vi "Save To TIFF.vi"(10 "Logging Cluster":T2 {"Exp params"."TSFrames" min=1 step=1; "Exp params"."TSfps" min=0.001 max=90.0 step=0.001 format="%_4g"}, 11 "img dst":T1) -> (3 "Image Out (duplicate)":T1)   [LabVIEW 2020]
uses:
  _controls/Logging Cluster.ctl
  _controls/Exp Params.ctl
  <vilib>/vision/Image Controls.llb/IMAQ Image.ctl
  _globals/OpticalPrime Controls.vi
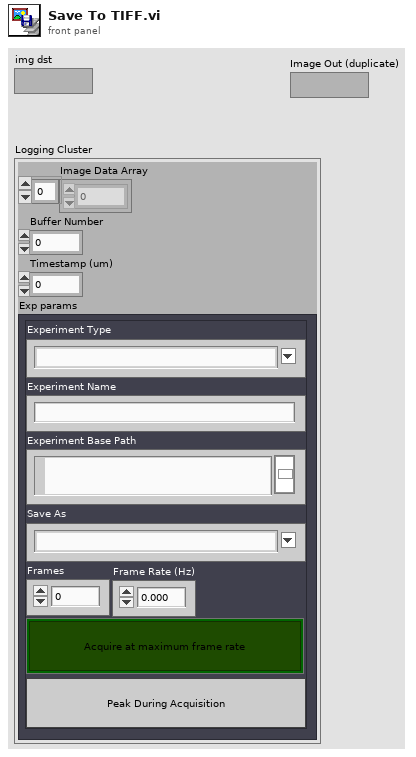
[diagram p1: front panel]
types:
  T1 = typedef "IMAQ Image.ctl" = refnum<image>
  T2 = typedef "Logging Cluster.ctl" = cluster{"Image Data Array":u8[], "Buffer Number":i32, "Timestamp (um)":u64, "Exp params":T3}
  T3 = typedef "Exp Params.ctl" = cluster{"Experiment Type":string, "Experiment Name":string, "ExpPath":path, "Save As":string, "TSFrames":i32, "TSfps":dbl, "Streaming":bool, "tdms ref":refnum<k34>, "frame #":i64, "Full Path":path, "PeakOnQueue":bool}
  T4 = enum16{"open", "replace", "create", "open or create", "replace or create", "replace or create with confirmation"}
  T5 = typedef "xiCam.ctl" = cluster{"Exposure Time (ms)":u32, "cam0 Session":T6, "Camera ROI":cluster{"Width":u32, "Height":u32, "Offset X":u32, "Offset Y":u32}, "Command":string}
  T6 = typedef "IMAQdx.ctl" = refnum<k21>
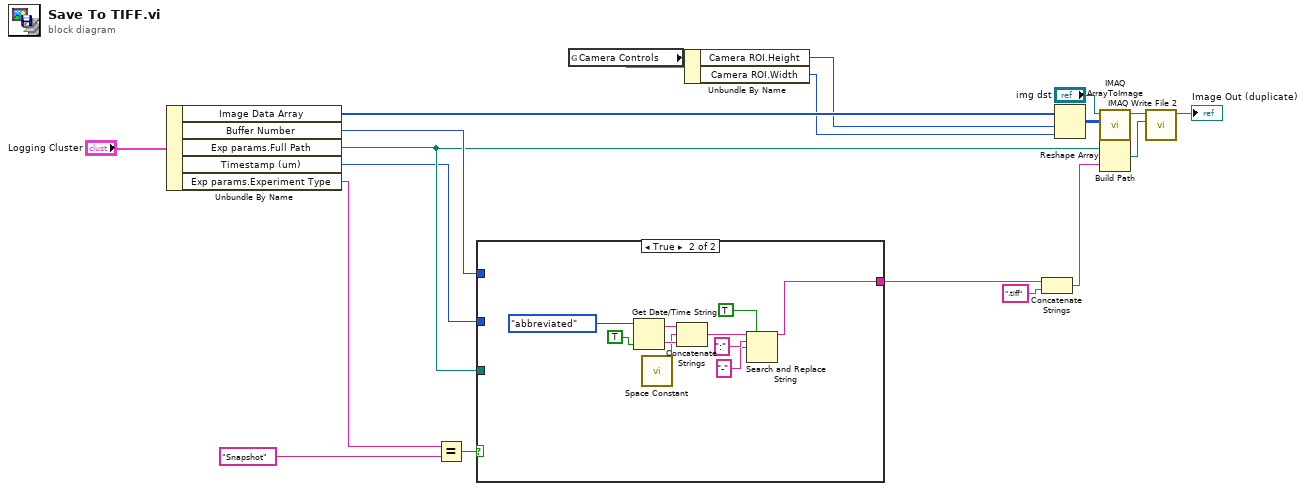
[diagram p0: block diagram]
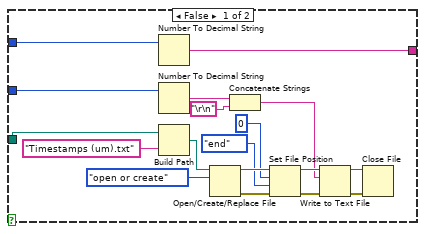
[diagram p2: hidden frame]
diagram:
  n1 = Unbundle By Name("Logging Cluster") -> ("Image Data Array"=w14:u8[], "Buffer Number"=w19:i32, "Exp params.Full Path"=w12:path, "Timestamp (um)"=w11:u64, "Exp params.Experiment Type"=w8:string)
  n2 = Equal?(x=w8, y="Snapshot" ("name or relative path")) -> (x = y?=w9:bool)
  n3 = case shown="True" w9 {
    tunnel: w19 -> [w37 _]
    tunnel: w12 -> [w33 _]
    tunnel: w11 -> [w27 _]
    tunnel: [w20 w38] -> w6
    frame False {
      n4 = Number To Decimal String(number=w37) -> (decimal integer string=w20:string)  [unwired: 1 in]
      n5 = Number To Decimal String(number=w27) -> (decimal integer string=w23:string)  [unwired: 1 in]
      n6 = Build Path(base path=w33, name or relative path="Timestamps (um).txt") -> (appended path=w32:path)
      n7 = Open/Create/Replace File(file path (use dialog)=w32, operation (0:open)=T4."open or create") -> (refnum out=w31:refnum<file>, error out=w35:errorcluster)  [unwired: 4 in, 1 out]
      n8 = Concatenate Strings(w23, "\r\n") -> (w21:string)
      n9 = Set File Position(offset (in bytes) (0)=i64 0, refnum=w31, from (0:start)=enum16{"start", "end", "current"}."end", error in=w35) -> (refnum out=w28:refnum<file>, error out=w25:errorcluster)
      n10 = Write to Text File(file (use dialog)=w28, text=w21, error in=w25) -> (refnum out=w26:refnum<file>, error out=w24:errorcluster)  [unwired: 1 in, 1 out]
      n11 = Close File(refnum=w26, error in=w24) -> ()  [unwired: 2 out]
    }
    frame True {
      n12 = Get Date/Time String(date format (0)=enum16{"short", "long", "abbreviated"}."abbreviated", want seconds? (F)=TRUE) -> (date string=w45:string, time string=w44:string)  [unwired: 1 in]
      n13 = call <vilib>:"Space Constant.vi"() -> ("String"=w43:string)
      n14 = Concatenate Strings(w45, w43, w44) -> (w42:string)
      n15 = Search and Replace String(replace all?=TRUE ("replace all? (F)"), input string=w42, search string=":", replace string="-" ("replace string (\"\")")) -> (result string=w38:string)  [unwired: 4 in, 3 out]
    }
  }
  n16 = global read "OpticalPrime Controls.vi" "Camera Controls"() -> (w3:T5)
  n17 = Unbundle By Name(w3) -> ("Camera ROI.Height"=w2:u32, "Camera ROI.Width"=w1:u32)
  n18 = Concatenate Strings(w6, ".tiff" ("string")) -> (w4:string)
  n19 = Reshape Array(w14, w2, w1) -> (w15:u8[][])
  n20 = call "IMAQ ArrayToImage"("Image Pixels (U8)"=w15, "Image"="img dst") -> ("Image Out"=w17:T1)  [unwired: 8 in, 1 out]
  n21 = Build Path(base path=w12, name or relative path=w4) -> (appended path=w16:path)
  n22 = call-poly "IMAQ Write File 2"("File Path"=w16, "Image"=w17) -> ("Image Out (duplicate)"=→"Image Out (duplicate)":T1)  [unwired: 8 in, 1 out]
